vi "IRDistance.vi"() -> ()   [LabVIEW 2017]
uses:
  <vilib>/Analysis/baseanly.llb/Mean (DBL).vi
  <vilib>/Analysis/NI_AALPro.lvlib
  <vilib>/Analysis/NI_AALBase.lvlib
panel:
  out "interpolation value":dbl format="%0.2f"
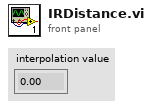
[diagram p1: front panel]
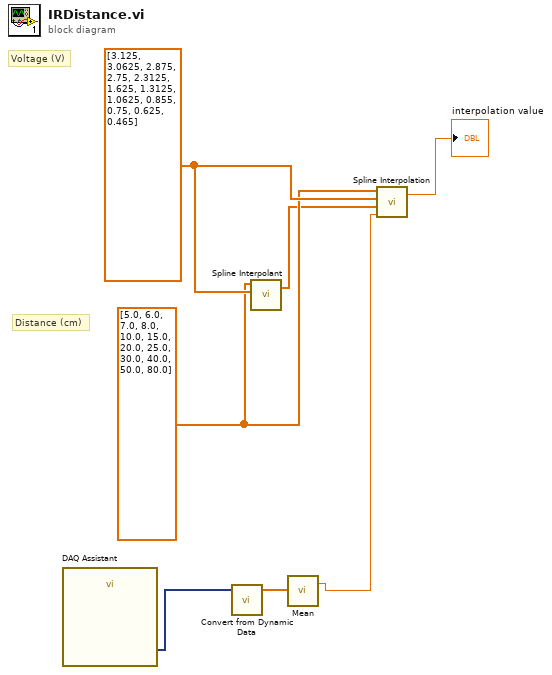
[diagram p0: block diagram]
diagram:
  w3 = dbl[] [5.0, 6.0, 7.0, 8.0, 10.0, 15.0, 20.0, 25.0, 30.0, 40.0, 50.0, 80.0] ("Array - Numeric")
  w7 = dbl[] [3.125, 3.0625, 2.875, 2.75, 2.3125, 1.625, 1.3125, 1.0625, 0.855, 0.75, 0.625, 0.465] ("Array - Numeric")
  # "Distance (cm)"
  # "Voltage (V)"
  n1 = call "DAQ Assistant"() -> ("data"=w6:dynamicdata)  [unwired: 16 in, 3 out]
  n2 = call "Convert from Dynamic Data"("Dynamic Data Type"=w6) -> ("Array"=w5:dbl[])  [unwired: 3 in]
  n3 = call <vilib>:"Spline Interpolant.vi"("X"=w7, "Y"=w3) -> ("Interpolant"=w2:dbl[])  [unwired: 2 in, 1 out]
  n4 = call-poly <vilib>:"Mean.vi"("X"=w5) -> ("mean"=w4:dbl)  [unwired: 1 out]
  n5 = call <vilib>:"Spline Interpolation.vi"("x value"=w4, "Interpolant"=w2, "X"=w7, "Y"=w3) -> ("interpolation value"=→"interpolation value":dbl)  [unwired: 1 out]
